vi "Check Disk Space Usage.vi"() -> ()   [LabVIEW 2020]
panel:
  in  "file path (use dialog)":path
  in  "Stop":bool
  out "Space Used Slide":dbl(slide) scale=0.0..100.0
  out "Space Used %":dbl
  out "free (Gb)":dbl
  out "total size (Gb)":dbl
  out "disk path":path
  out "error out":errorcluster
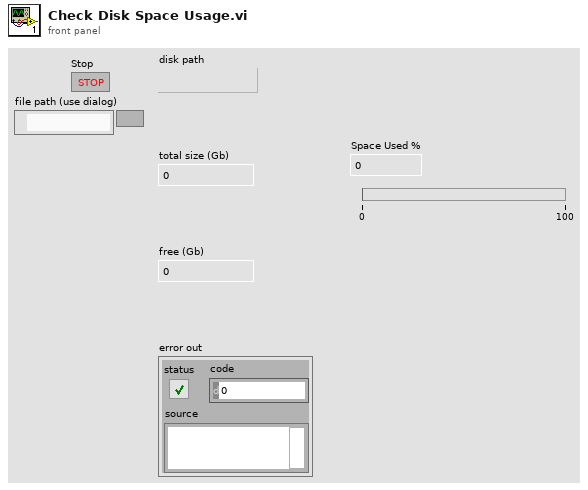
[diagram p1: front panel]
types:
  T1 = enum16{"open", "replace", "create", "open or create", "replace or create", "replace or create with confirmation"}
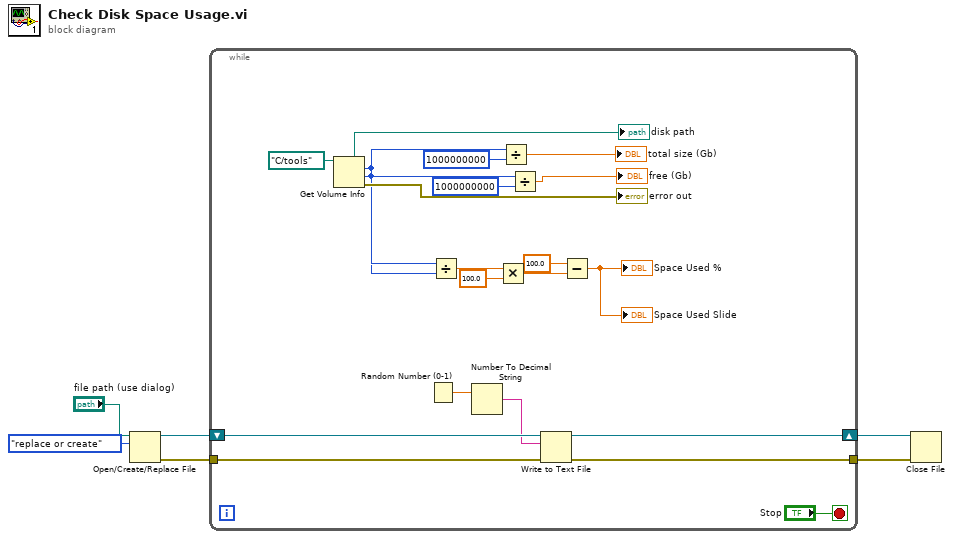
[diagram p0: block diagram]
diagram:
  n1 = Open/Create/Replace File(file path (use dialog)="file path (use dialog)", operation (0:open)=T1."replace or create") -> (refnum out=w6:refnum<file>, error out=w5:errorcluster)  [unwired: 4 in, 1 out]
  n2 = while {
    tunnel: w5 -> [w12]
    tunnel: [w11] -> w2
    shift-right: [w9] -> w1
    shift-left: w6 -> [w10]
    stop <- "Stop" stop-if-true
    n3 = Get Volume Info(11:path "C:/tools" ("path")) -> (0:→"error out":errorcluster, 1:w23:i64, 2:w22:i64, 5:→"disk path":path)  [unwired: 1 in, 2 out]
    n4 = Random Number (0-1)() -> (number: 0 to 1=w8:dbl)
    n5 = Divide(x=w23, y=w22) -> (x/y=w24:dbl)
    n6 = Number To Decimal String(number=w8) -> (decimal integer string=w7:string)  [unwired: 1 in]
    n7 = Multiply(x=w24, y=100.0) -> (x*y=w20:dbl)
    n8 = Divide(x=w22, y=i64 1000000000) -> (x/y=→"total size (Gb)":dbl)
    n9 = Divide(x=w23, y=i64 1000000000) -> (x/y=→"free (Gb)":dbl)
    n10 = Write to Text File(file (use dialog)=w10, text=w7, error in=w12) -> (refnum out=w9:refnum<file>, error out=w11:errorcluster)  [unwired: 1 in, 1 out]
    n11 = Subtract(x=100.0 ("y"), y=w20) -> (x-y=→"Space Used %" →"Space Used Slide":dbl)
  }
  n12 = Close File(refnum=w1, error in=w2) -> ()  [unwired: 2 out]
